vi "Get Settings.vi"(11 "Configuration in":refnum<class "Configuration.lvclass">) -> (2 "settings":T1, 3 "Configuration out":refnum<class "Configuration.lvclass">)   [LabVIEW 2017, in "Data Sharing Framework Engine.lvlib" / "Configuration.lvclass"]
uses:
  Configuration.lvclass
  Configuration/1.0.0/Public/Controls/DSF Settings Info.ctl
  Configuration.lvclass/Configuration.ctl
  Configuration/1.0.0/Data Sharing Framework Configuration.lvlib
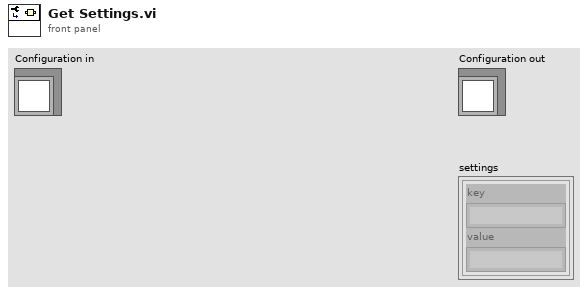
[diagram p1: front panel]
types:
  T1 = typedef "Data Sharing Framework Configuration.lvlib/DSF Settings Info.ctl" = cluster{"key":string, "value":string}[]
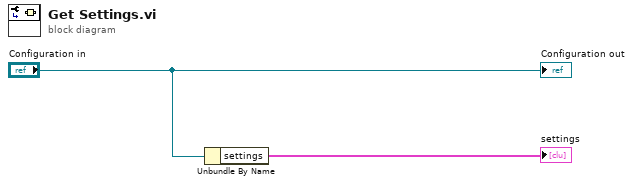
[diagram p0: block diagram]
diagram:
  n1 = Unbundle By Name("Configuration in") -> ("settings"=→"settings":T1)
  "Configuration out" <- "Configuration in"
